vi "AlGaAs_wait_SL.vi"(2 "Debug Mode":bool, 3 "Elapsed Time(s)":dbl, 4 "State":enum16{"Edit", "Start", "Run", "End", "Idle"}(ring), 5 "Argument List In":string[](array[string])) -> (0 "Status Out":string, 1 "Argument List Out":string[](array[string]))   [LabVIEW 2011]
panel:
  in  "Al2 flow (sccm)":dbl
  in  "Ga1 flow (sccm)":dbl
  out "tphase(s)":dbl[](array[numeric])
  out "nstep":dbl
  out "phase":i32
  out "done":bool
  in  "t1 wait (s)":dbl
  in  "t1 flow (s)":dbl
  in  "Al1 flow (sccm)":dbl
  in  "nPeriods":dbl
  out "tTotal(s)":dbl
  out "tPeriod(s)":dbl
  in  "t2 wait (s)":dbl
  in  "t2 flow (s)":dbl
  in  "Ga2 flow (sccm)":dbl
  in  "Cancel":bool
  in  "OK":bool
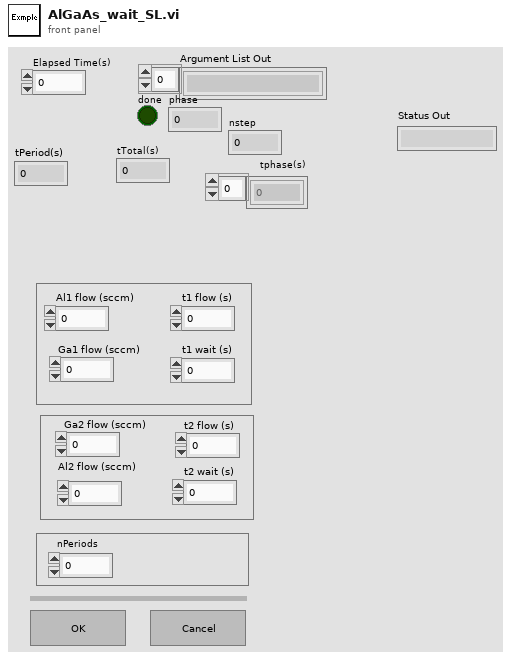
[diagram p1: front panel]
types:
  T1 = enum16{"Discrete", "Continuous", "Instantaneous"}
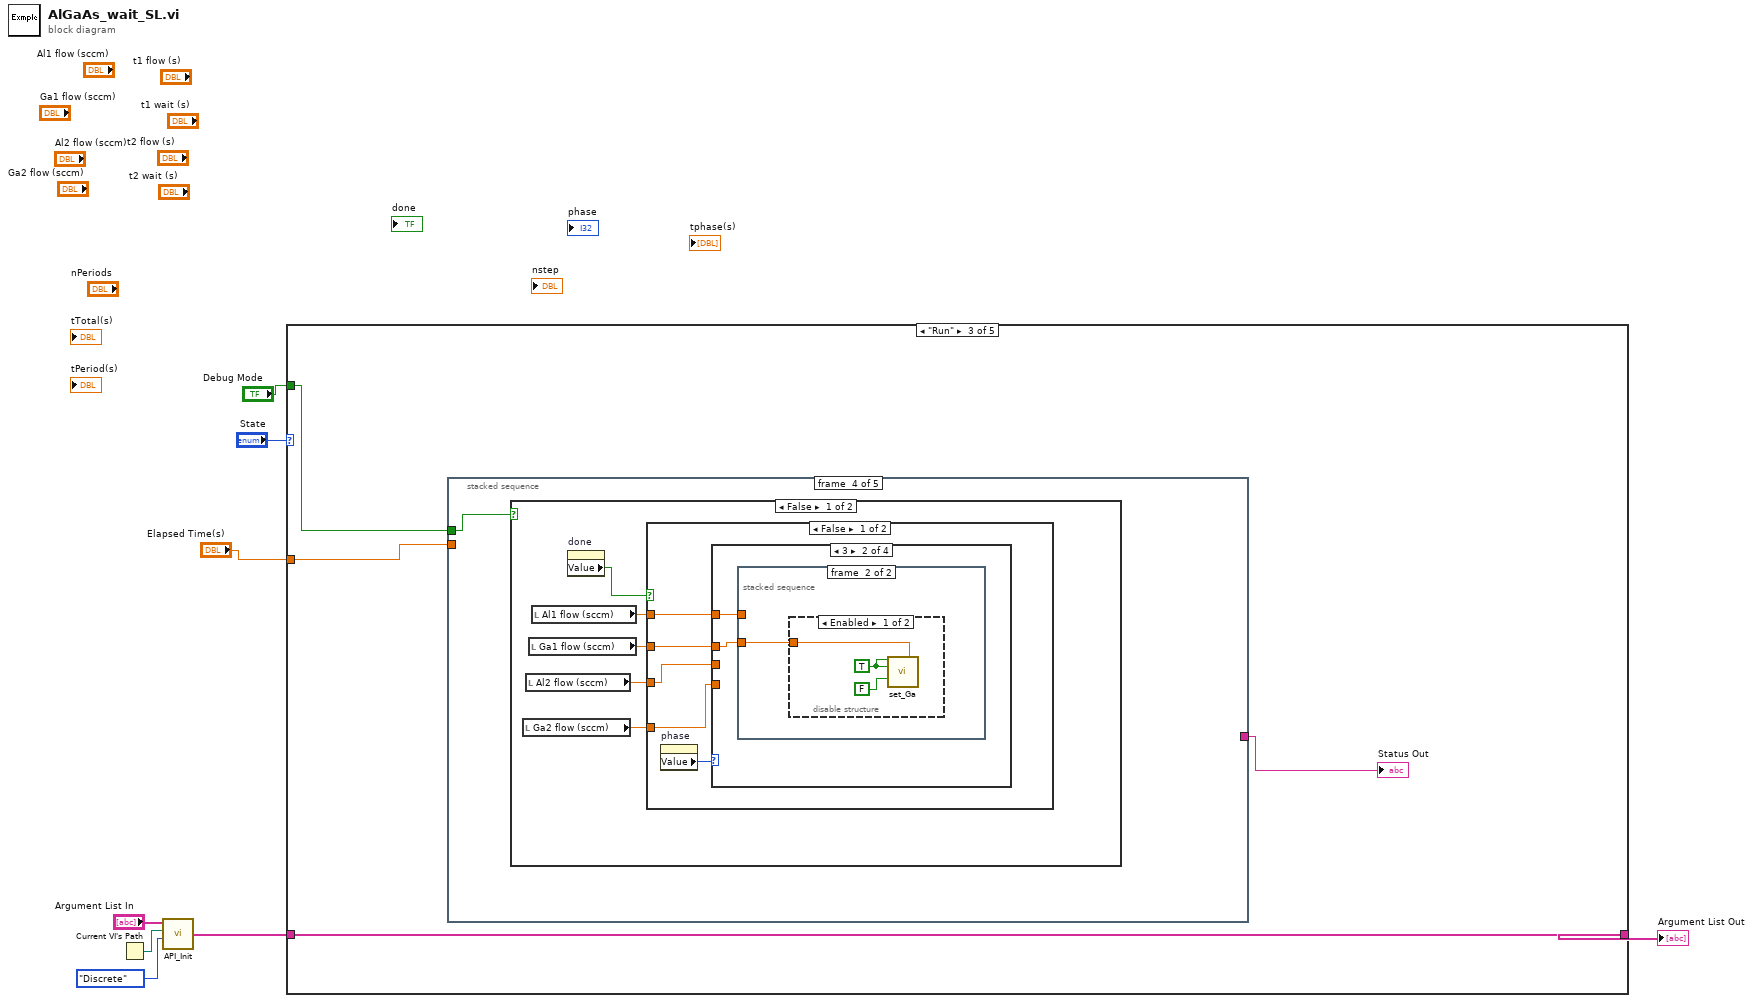
[diagram p0: block diagram]
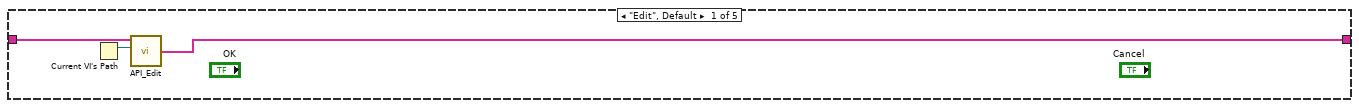
[diagram p2: hidden frame]
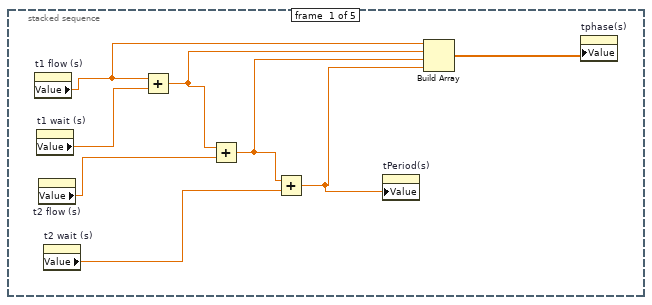
[diagram p4: hidden frame]
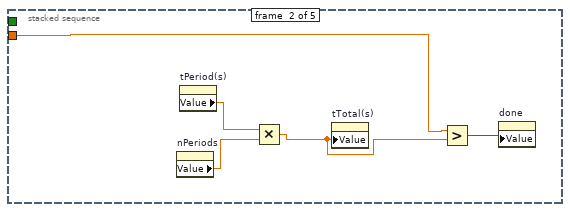
[diagram p5: hidden frame]
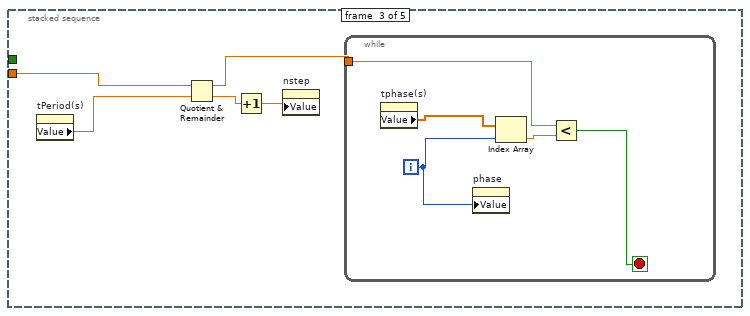
[diagram p6: hidden frame]
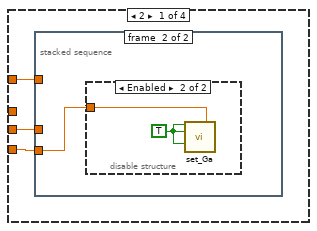
[diagram p7: hidden frame]
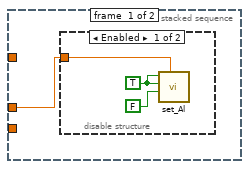
[diagram p8: hidden frame]
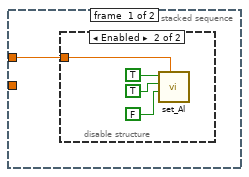
[diagram p11: hidden frame]
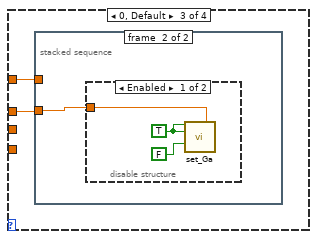
[diagram p14: hidden frame]
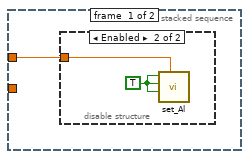
[diagram p15: hidden frame]
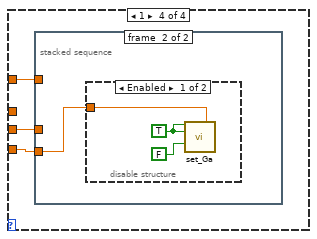
[diagram p18: hidden frame]
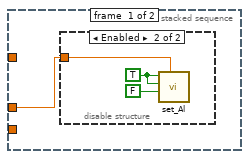
[diagram p19: hidden frame]
diagram:
  n1 = Current VI's Path() -> (path=w5:path)
  n2 = call "API_Init.vi"("API Mode"=T1."Discrete", "VI Path"=w5, "Argument List In"="Argument List In") -> ("Argument List Out"=w6:string[])  [unwired: 1 in]
  n3 = case shown="\"Run\"" "State" {
    tunnel: [w9 w12 w16 w133 w134] -> w2
    tunnel: w6 -> [w11 w12 w16 w133 w134]
    tunnel: "Debug Mode" -> [_ _ w14 _ _]
    tunnel: "Elapsed Time(s)" -> [_ _ w15 _ _]
    frame "Edit", Default {
      n4 = Current VI's Path() -> (path=w10:path)
      n5 = call "API_Edit.vi"("VI Path"=w10, "Argument List In"=w11) -> ("Argument List Out"=w9:string[])  [unwired: 2 in]
    }
    frame "Start" {
    }
    frame "Run" {
      n6 = stacked-sequence {
        tunnel: w15 -> [_ w27 w34 _ _]
        tunnel: w14 -> [_ _ _ w40 _]
        tunnel: [_ _ _ _ w102] -> w13
        frame #0 {
          n7 = property on="t1 flow (s)" class="DigNum (strict)"() -> ("Value"=w23:dbl)  [unwired: 2 in, 2 out]
          n8 = property on="t1 wait (s)" class="DigNum (strict)"() -> ("Value"=w24:dbl)  [unwired: 2 in, 2 out]
          n9 = property on="t2 flow (s)" class="DigNum (strict)"() -> ("Value"=w21:dbl)  [unwired: 2 in, 2 out]
          n10 = property on="t2 wait (s)" class="DigNum (strict)"() -> ("Value"=w20:dbl)  [unwired: 2 in, 2 out]
          n11 = Add(x=w23, y=w24) -> (x+y=w22:dbl)
          n12 = Add(x=w22, y=w21) -> (x+y=w19:dbl)
          n13 = Add(x=w19, y=w20) -> (x+y=w18:dbl)
          n14 = property on="tPeriod(s)" class="DigNum (strict)"("Value"=w18) -> ()  [unwired: 2 in, 2 out]
          n15 = Build Array(w23, w22, w19, w18) -> (w17:dbl[])
          n16 = property on="tphase(s)" class="Arr (strict)"("Value"=w17) -> ()  [unwired: 2 in, 2 out]
        }
        frame #1 {
          n17 = property on="nPeriods" class="DigNum (strict)"() -> ("Value"=w28:dbl)  [unwired: 2 in, 2 out]
          n18 = property on="tPeriod(s)" class="DigNum (strict)"() -> ("Value"=w29:dbl)  [unwired: 2 in, 2 out]
          n19 = Multiply(x=w29, y=w28) -> (x*y=w26:dbl)
          n20 = property on="tTotal(s)" class="DigNum (strict)"("Value"=w26) -> ()  [unwired: 2 in, 2 out]
          n21 = Greater?(x=w27, y=w26) -> (0:w25:bool)
          n22 = property on="done" class="Bool (strict)"("Value"=w25) -> ()  [unwired: 2 in, 2 out]
        }
        frame #2 {
          n23 = property on="tPeriod(s)" class="DigNum (strict)"() -> ("Value"=w33:dbl)  [unwired: 2 in, 2 out]
          n24 = Quotient & Remainder(x=w34, y=w33) -> (x-y*floor(x/y)=w32:dbl, floor(x/y)=w31:dbl)
          n25 = Increment(x=w31) -> (x+1=w30:dbl)
          n26 = property on="nstep" class="DigNum (strict)"("Value"=w30) -> ()  [unwired: 2 in, 2 out]
          n27 = while {
            tunnel: w32 -> [w38]
            i -> [w36]
            stop <- w35 stop-if-true
            n28 = property on="tphase(s)" class="Arr (strict)"() -> ("Value"=w39:dbl[])  [unwired: 2 in, 2 out]
            n29 = property on="phase" class="DigNum (strict)"("Value"=w36) -> ()  [unwired: 2 in, 2 out]
            n30 = Index Array(array=w39, index=w36) -> (element=w37:dbl)
            n31 = Less?(x=w38, y=w37) -> (x < y?=w35:bool)
          }
        }
        frame #3 {
          n32 = case shown="False" w40 {
            frame False {
              n33 = local read "Ga2 flow (sccm)"() -> (w43:dbl)
              n34 = local read "Al2 flow (sccm)"() -> (w41:dbl)
              n35 = local read "Ga1 flow (sccm)"() -> (w42:dbl)
              n36 = local read "Al1 flow (sccm)"() -> (w45:dbl)
              n37 = property on="done" class="Bool (strict)"() -> ("Value"=w44:bool)  [unwired: 2 in, 2 out]
              n38 = case shown="False" w44 {
                tunnel: w45 -> [w50 w93]
                tunnel: w43 -> [w48 _]
                tunnel: w42 -> [w47 _]
                tunnel: w41 -> [w46 _]
                frame False {
                  n39 = property on="phase" class="DigNum (strict)"() -> ("Value"=w49:i32)  [unwired: 2 in, 2 out]
                  n40 = case shown="3" w49 {
                    tunnel: w50 -> [w53 w62 w73 w83]
                    tunnel: w48 -> [w52 _ _ w82]
                    tunnel: w47 -> [_ w61 w72 _]
                    tunnel: w46 -> [w51 _ _ w81]
                    frame 2 {
                      n41 = stacked-sequence {
                        tunnel: w53 -> [_ _]
                        tunnel: w52 -> [_ w58]
                        tunnel: w51 -> [w54 _]
                        frame #0 {
                          n42 = disable-structure shown="Enabled" {
                            disable-tunnel: w54 -> [w55 _]
                            frame Enabled {
                              w57 = TRUE ("Ga Active")
                              n43 = call "set_Al.vi"("Aluminum Flow"=w55, "Al Run"=FALSE, "Al Bubbler"=w57, "Al Active"=w57) -> ()  [unwired: 6 in]
                            }
                            frame Disabled {
                            }
                          }
                        }
                        frame #1 {
                          n44 = disable-structure shown="Enabled" {
                            disable-tunnel: w58 -> [_ w60]
                            frame Disabled {
                            }
                            frame Enabled {
                              w59 = TRUE ("Ga Active")
                              n45 = call "set_Ga.vi"("Ga Active"=w59, "Ga Flow 1"=w60, "Ga Bubbler"=w59, "Ga Run"=w59) -> ()  [unwired: 12 in]
                            }
                          }
                        }
                      }
                    }
                    frame 3 {
                      n46 = stacked-sequence {
                        tunnel: w62 -> [w63 _]
                        tunnel: w61 -> [_ w68]
                        frame #0 {
                          n47 = disable-structure shown="Enabled" {
                            disable-tunnel: w63 -> [_ w64]
                            frame Disabled {
                            }
                            frame Enabled {
                              n48 = call "set_Al.vi"("Aluminum Flow"=w64, "Al Run"=FALSE, "Al Bubbler"=TRUE, "Al Active"=TRUE) -> ()  [unwired: 6 in]
                            }
                          }
                        }
                        frame #1 {
                          n49 = disable-structure shown="Enabled" {
                            disable-tunnel: w68 -> [w69 _]
                            frame Enabled {
                              w70 = TRUE ("Ga Active")
                              n50 = call "set_Ga.vi"("Ga Active"=w70, "Ga Flow 1"=w69, "Ga Bubbler"=w70, "Ga Run"=FALSE) -> ()  [unwired: 4 in, 8 out]
                            }
                            frame Disabled {
                            }
                          }
                        }
                      }
                    }
                    frame 0, Default {
                      n51 = stacked-sequence {
                        tunnel: w73 -> [w74 _]
                        tunnel: w72 -> [_ w77]
                        frame #0 {
                          n52 = disable-structure shown="Enabled" {
                            disable-tunnel: w74 -> [_ w76]
                            frame Disabled {
                            }
                            frame Enabled {
                              w75 = TRUE ("Al Active")
                              n53 = call "set_Al.vi"("Aluminum Flow"=w76, "Al Run"=w75, "Al Bubbler"=w75, "Al Active"=w75) -> ()  [unwired: 6 in]
                            }
                          }
                        }
                        frame #1 {
                          n54 = disable-structure shown="Enabled" {
                            disable-tunnel: w77 -> [w78 _]
                            frame Enabled {
                              w79 = TRUE ("Ga Active")
                              n55 = call "set_Ga.vi"("Ga Active"=w79, "Ga Flow 1"=w78, "Ga Bubbler"=w79, "Ga Run"=FALSE) -> ()  [unwired: 4 in, 8 out]
                            }
                            frame Disabled {
                            }
                          }
                        }
                      }
                    }
                    frame 1 {
                      n56 = stacked-sequence {
                        tunnel: w82 -> [_ w88]
                        tunnel: w83 -> [_ _]
                        tunnel: w81 -> [w84 _]
                        frame #0 {
                          n57 = disable-structure shown="Enabled" {
                            disable-tunnel: w84 -> [_ w86]
                            frame Disabled {
                            }
                            frame Enabled {
                              w85 = TRUE ("Al Bubbler")
                              n58 = call "set_Al.vi"("Aluminum Flow"=w86, "Al Run"=FALSE, "Al Bubbler"=w85, "Al Active"=w85) -> ()  [unwired: 6 in]
                            }
                          }
                        }
                        frame #1 {
                          n59 = disable-structure shown="Enabled" {
                            disable-tunnel: w88 -> [w89 _]
                            frame Enabled {
                              w90 = TRUE ("Ga Active")
                              n60 = call "set_Ga.vi"("Ga Active"=w90, "Ga Flow 1"=w89, "Ga Bubbler"=w90, "Ga Run"=FALSE) -> ()  [unwired: 4 in, 8 out]
                            }
                            frame Disabled {
                            }
                          }
                        }
                      }
                    }
                  }
                }
                frame True {
                  n61 = stacked-sequence {
                    tunnel: w93 -> [w94 _]
                    tunnel: [_ w98] -> w92
                    frame #0 {
                      n62 = disable-structure shown="Enabled" {
                        disable-tunnel: w94 -> [_ w97]
                        frame Disabled {
                        }
                        frame Enabled {
                          w96 = TRUE ("Al Active")
                          n63 = call "set_Al.vi"("Aluminum Flow"=w97, "Al Run"=FALSE, "Al Bubbler"=w96, "Al Active"=w96) -> ()  [unwired: 6 in]
                        }
                      }
                    }
                    frame #1 {
                      n64 = disable-structure shown="Enabled" {
                        disable-tunnel: w98 -> [w99 _]
                        frame Enabled {
                          w100 = TRUE ("Ga Active")
                          n65 = call "set_Ga.vi"("Ga Active"=w100, "Ga Flow 1"=w99, "Ga Bubbler"=w100, "Ga Run"=FALSE) -> ()  [unwired: 4 in, 8 out]
                        }
                        frame Disabled {
                        }
                      }
                    }
                  }
                }
              }
            }
            frame True {
            }
          }
        }
        frame #4 {
          n66 = property on="done" class="Bool (strict)"() -> ("Value"=w103:bool)  [unwired: 2 in, 2 out]
          n67 = case shown="True" w103 {
            tunnel: [w104 w132] -> w102
            frame False {
              n68 = property on="phase" class="DigNum (strict)"() -> ("Value"=w111:i32)  [unwired: 2 in, 2 out]
              n69 = case shown="0, Default" w111 {
                tunnel: [w114 "wait (Ga)" w121 "wait (Al)"] -> w110
                frame 2 {
                  n70 = local read "Ga2 flow (sccm)"() -> (w113:dbl)
                  n71 = Format Into String(format string="%4.2f", w113) -> (resulting string=w117:string)  [unwired: 2 in, 1 out]
                  n72 = Concatenate Strings("Ga(" ("string"), w117, "sccm)" ("string")) -> (w114:string)
                }
                frame 3 {
                }
                frame 0, Default {
                  n73 = local read "Al1 flow (sccm)"() -> (w120:dbl)
                  n74 = Format Into String(format string="%4.1f", w120) -> (resulting string=w123:string)  [unwired: 2 in, 1 out]
                  n75 = Concatenate Strings("Al(" ("string"), w123, "sccm)" ("string")) -> (w121:string)
                }
                frame 1 {
                }
              }
              n76 = property on="nstep" class="DigNum (strict)"() -> ("Value"=w112:dbl)  [unwired: 2 in, 2 out]
              n77 = Format Into String(format string="%3.0f", w112) -> (resulting string=w107:string)  [unwired: 2 in, 1 out]
              n78 = Concatenate Strings("Period " ("string"), w107) -> (w105:string)
              n79 = Concatenate Strings(w105, ", " ("string"), w110) -> (w104:string)
            }
            frame True {
              n80 = property on="nPeriods" class="DigNum (strict)"() -> ("Value"=w127:dbl)  [unwired: 2 in, 2 out]
              n81 = Format Into String(format string="%3.0f", w127) -> (resulting string=w128:string)  [unwired: 2 in, 1 out]
              n82 = Concatenate Strings("done after", w128, " periods" ("string")) -> (w132:string)
            }
          }
        }
      }
      "Status Out" <- w13
    }
    frame "End" {
    }
    frame "Idle" {
    }
  }
  "Argument List Out" <- w2
